vi "scan2d_check_stop_queue.vi"(8 "error in (no error)":errorcluster, 11 "scan_panel in":refnum<class "scan_2d.lvclass">) -> (0 "error out":errorcluster, 2 "stop?":bool, 3 "scan_panel out":refnum<class "scan_2d.lvclass">)   [LabVIEW 2015, in "scan_2d.lvclass"]
uses:
  scan_2d.lvclass
  scan_2d.lvclass/scan_2d.ctl
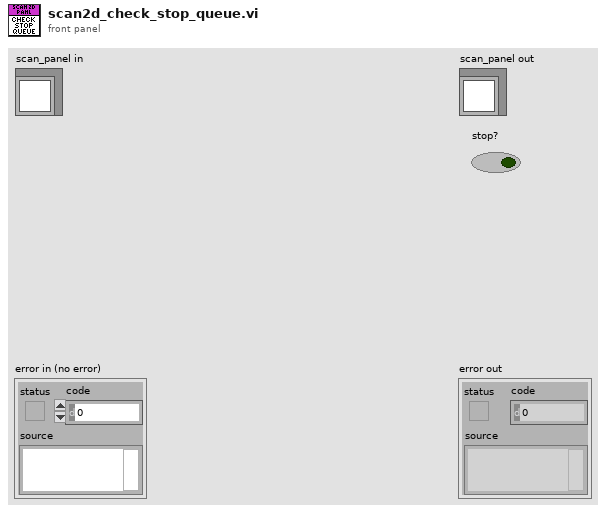
[diagram p1: front panel]
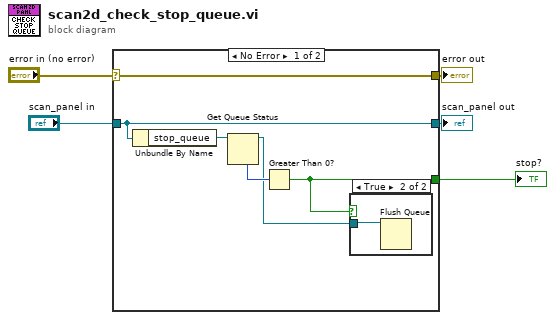
[diagram p0: block diagram]
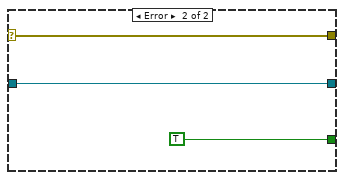
[diagram p3: hidden frame]
diagram:
  n1 = case shown="No Error" "error in (no error)" {
    selector: "error in (no error)" -> [w11 w15]
    tunnel: [w11 w15] -> w4
    tunnel: [w10 w14] -> w2
    tunnel: "scan_panel in" -> [w10 w14]
    tunnel: [w7 TRUE] -> w1
    frame No Error {
      n2 = Unbundle By Name(w10) -> ("stop_queue"=w9:refnum<queue>)
      n3 = Get Queue Status(queue=w9) -> (queue out=w6:refnum<queue>, # elements in queue=w8:i32)  [unwired: 2 in, 6 out]
      n4 = Greater Than 0?(x=w8) -> (x > 0?=w7:bool)
      n5 = case shown="True" w7 {
        tunnel: w6 -> [_ w12]
        frame False {
        }
        frame True {
          n6 = Flush Queue(queue=w12) -> ()  [unwired: 1 in, 3 out]
        }
      }
    }
    frame Error {
    }
  }
  "error out" <- w4
  "scan_panel out" <- w2
  "stop?" <- w1
